vi "AO Array Add or Remove.vi"(8 "error in (no error)":errorcluster, 10 "Size":i32, 11 "AO Channels in":T1 {"Phase" format="%#_3g"; "Frequency" min=0.0001 max=200000.0 format="%#_6p"; "Offset" format="%#_6p"; "Amplitude" min=0.0 max=10.0 format="%#_6p"}) -> (0 "error out":errorcluster, 3 "AO Channels out":T1 {"Phase" format="%#_3g"; "Frequency" min=0.0001 max=200000.0 format="%#_6p"; "Offset" format="%#_6p"; "Amplitude" min=0.0 max=10.0 format="%#_6p"})   [LabVIEW 2019, in "Instrument.Lockin.lvlib" / "Instrument.DAQ.lvclass"]
uses:
  Instrument.DAQ.lvclass
  Typedefs/AO.Channel--Cluster--Array.ctl
  Typedefs/AO.Channel--Cluster.ctl
  Typedefs/AO.Channel.Function--Enum.ctl
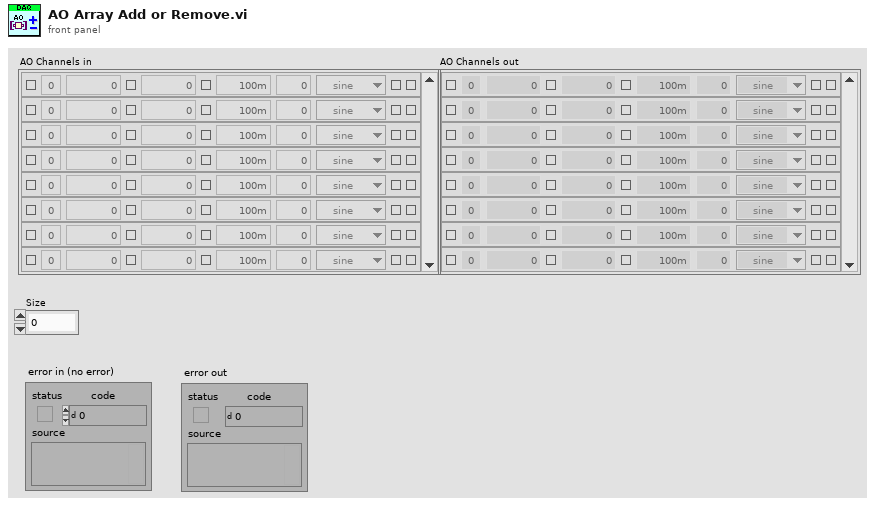
[diagram p1: front panel]
types:
  T1 = typedef "Instrument.Lockin.lvlib/Instrument.DAQ.lvclass/AO.Channel--Cluster--Array.ctl" = T2[]
  T2 = typedef "Instrument.Lockin.lvlib/Instrument.DAQ.lvclass/AO.Channel--Cluster.ctl" = cluster{"Enable?":bool, "Channel":i32, "Amplitude":dbl, "Offset":dbl, "Frequency":dbl, "Phase":dbl, "Function":T3, "Sweeping?":bool, "Limit AC":bool, "Limit DC?":bool, "Duty Cycle":bool}
  T3 = typedef "Instrument.Lockin.lvlib/Instrument.DAQ.lvclass/AO.Channel.Function--Enum.ctl" = enum16{"sine", "square", "triangle", "saw"}
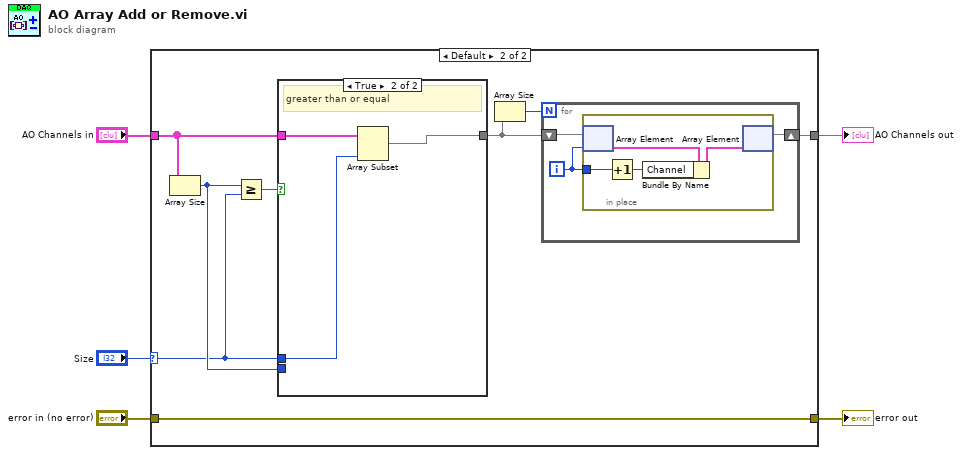
[diagram p0: block diagram]
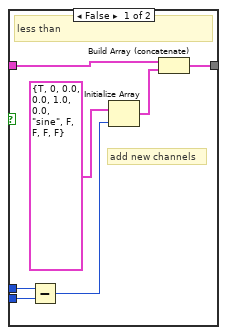
[diagram p3: hidden frame]
diagram:
  n1 = case shown="Default" "Size" {
    selector: "Size" -> [_ w13]
    tunnel: [w7 w12] -> w4
    tunnel: "AO Channels in" -> [w7 w8]
    tunnel: [w6 w11] -> w2
    tunnel: "error in (no error)" -> [w6 w11]
    frame 0 {
    }
    frame Default {
      n2 = Array Size(array=w8) -> (size(s)=w15:i32)
      n3 = Greater Or Equal?(x=w15, y=w13) -> (x >= y?=w14:bool)
      n4 = case shown="True" w14 {
        tunnel: w8 -> [w17 w25]
        tunnel: w13 -> [w20 w24]
        tunnel: [w21 w23] -> w10
        tunnel: w15 -> [w19 _]
        frame False {
          # "add new channels"
          # "less than"
          n5 = Subtract(x=w20, y=w19) -> (x-y=w18:i32)
          n6 = Initialize Array(T2 {"Enable?"=TRUE, "Channel"=0, "Amplitude"=0.0, "Offset"=0.0, "Frequency"=1.0, "Phase"=0.0, "Function"=enum."sine", "Sweeping?"=FALSE, "Limit AC"=FALSE, "Limit DC?"=FALSE, "Duty Cycle"=FALSE} ("AO"), w18) -> (w22:T2[])
          n7 = Build Array (concatenate)(w17, w22) -> (w21:T1)
        }
        frame True {
          # "greater than or equal"
          n8 = Array Subset(array=w25, length=w24) -> (w23:T1)  [unwired: 1 in]
        }
      }
      n9 = Array Size(array=w10) -> (size(s)=w9:i32)
      n10 = for {
        N: w9 -> [_]
        shift-right: [w26] -> w12
        shift-left: w10 -> [w28]
        i -> [w27]
        n11 = in-place {
          in-place-border: w27 -> [w31]
          n12 = in-place-array #1(w28, w27) -> (w30:T2)
          n13 = Increment(x=w31) -> (x+1=w32:i32)
          n14 = Bundle By Name(cluster=w30, "Channel"=w32) -> (w29:T2)
          n15 = in-place-array #1(w29) -> (w26:T1)  [unwired: 1 out]
        }
      }
    }
  }
  "AO Channels out" <- w4
  "error out" <- w2
